vi "Create Pulse Waveform.vi"(8 "error in (no error)":errorcluster, 11 "RFSoC Driver in":refnum<class "RFSoC Driver.lvclass">) -> (0 "error out":errorcluster, 2 "Array - Numeric":dbl[](array[numeric]), 3 "RFSoC Driver out":refnum<class "RFSoC Driver.lvclass">)   [LabVIEW 2020, in "RFSoC Driver.lvclass"]
uses:
  RFSoC Driver.lvclass
  PulseEcho/PulsedFieldEcho/Create_Pulse/Create_waveform/build_waveform.lvclass
panel:
  out "Waveform Graph":dbl[](graph)
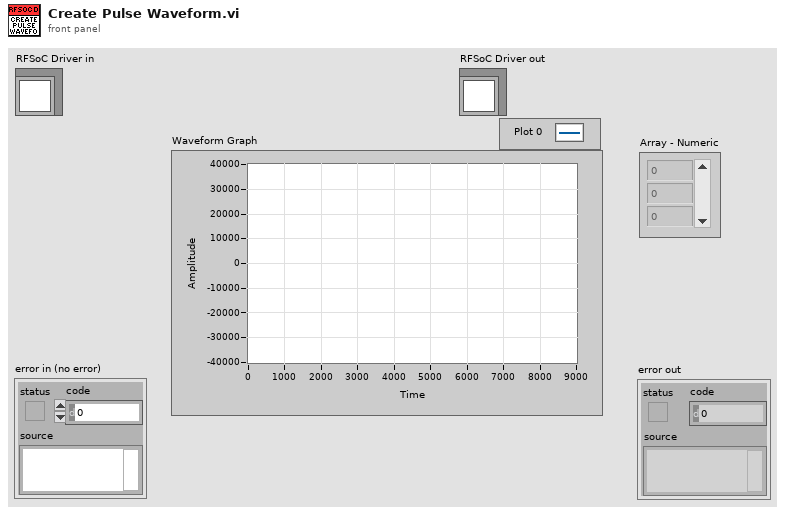
[diagram p1: front panel]
types:
  T1 = typedef "Pulse Parameters.ctl" = cluster{"clock rate":dbl, "Frequency":dbl, "NWaves":i32, "standard deviation":dbl, "Amplitude":dbl, "Mode":enum16{"Sine", "Pulse"}}
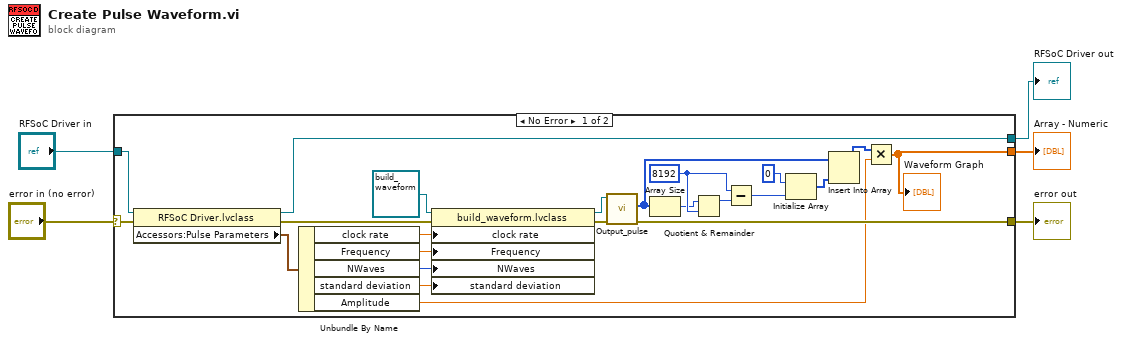
[diagram p0: block diagram]
diagram:
  n1 = case shown="No Error" "error in (no error)" {
    selector: "error in (no error)" -> [w23 w30]
    tunnel: [w13 w30] -> w4
    tunnel: [w9 w29] -> w2
    tunnel: "RFSoC Driver in" -> [w10 w29]
    tunnel: [w12 _] -> w1
    frame No Error {
      w17 = 8192
      n2 = property class="RFSoC Driver.lvclass"(reference=w10, error in=w23) -> (reference out=w9:refnum<class "RFSoC Driver.lvclass">, error out=w11:errorcluster, "Accessors:Pulse Parameters"=w8:T1)
      n3 = Unbundle By Name(w8) -> ("clock rate"=w28:dbl, "Frequency"=w27:dbl, "NWaves"=w26:i32, "standard deviation"=w25:dbl, "Amplitude"=w7:dbl)
      n4 = property class="build_waveform.lvclass"(reference=refnum<class "build_waveform.lvclass"> refnum ("build_waveform.lvclass"), error in=w11, "clock rate"=w28, "Frequency"=w27, "NWaves"=w26, "standard deviation"=w25) -> (reference out=w14:refnum<class "build_waveform.lvclass">, error out=w15:errorcluster)
      n5 = call-dynamic "Output_pulse.vi"("error in (no error)"=w15, "build_waveform in"=w14) -> ("error out"=w13:errorcluster, "Array"=w22:i8[])  [unwired: 7 in, 1 out]
      n6 = Array Size(array=w22) -> (size(s)=w16:i32)
      n7 = Quotient & Remainder(x=w16, y=w17) -> (x-y*floor(x/y)=w18:i32)  [unwired: 1 out]
      n8 = Subtract(x=w17, y=w18) -> (x-y=w21:i32)
      n9 = Initialize Array(i16 0 ("element"), w21) -> (w20:i16[])
      n10 = Insert Into Array(array=w22, new element=w20) -> (w6:i8[])  [unwired: 1 in]
      n11 = Multiply(x=w6, y=w7) -> (x*y=w12:dbl[])
      "Waveform Graph" <- w12
    }
    frame Error {
    }
  }
  "error out" <- w4
  "RFSoC Driver out" <- w2
  "Array - Numeric" <- w1
